vi "LVDimInterface.dim_dispatcher.vi"(2 "start":refnum<k4>, 4 "stop":refnum<k4>) -> ()   [LabVIEW 2014, in "LVDimInterface.lvlib"]
doc: "This VI should only be used, when using the DIMWrapper interface in polling mode. This VI must be started prior to any other DIM VIs. This VI must only exist once per execution system.\n\nHistory: 22-FEB-2006, Dietrich Beck\n\nCopyright (C)\nGesellschaft für Schwerionenforschung, GSI\nPlanckstr. 1\n64291 Darmstadt\nGermany\n\nContact: D.Beck@gsi.de \n\nThis program is free software; you can redistribute it and/or modify it under the terms of the \nGNU General Public License as published by the Free Software Foundation; either version 2 of the license, or (at your option) any later version.\n\nThis program is distributed in the hope that it will be useful, but WITHOUT ANY WARRANTY; without even the implied warranty of MERCHANTABILITY or FITNESS FOR A PARTICULAR PURPOSE. See the GNU General License for more details (http://www.gnu.org).\n\nGesellschaft für Schwerionenforschung, GSI\nPlanckstr. 1, 64291 Darmstadt, Germany\nFor all questions and ideas contact D. Beck.\nLast update: 16-DEC-2005"
uses:
  LVDimInterface.lvlib
  LVDimInterface.queue type.ctl
  LVDimInterface.notifier type.ctl
  bin/libDimWrapper.dll
  bin/libDimWrapper.so
  bin/libDimWrapperSPL.dll
panel:
  out "error out":errorcluster
  out "pollingMode":bool
  in  "notifierRef":T1
  out "loopCounter":i32
  in  "queueRef":T2
  out "nOfReceived":i32
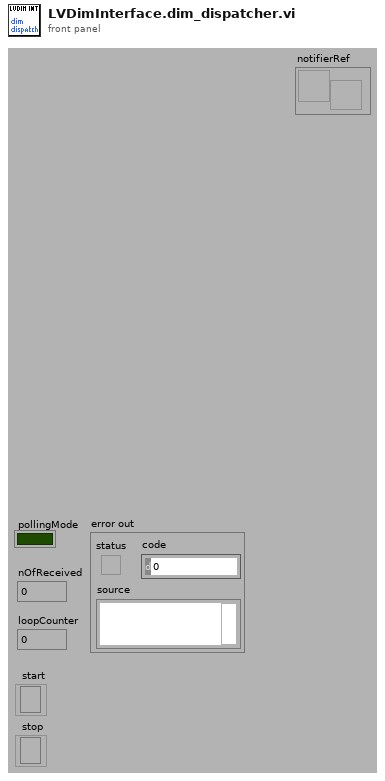
[diagram p1: front panel]
types:
  T1 = typedef "LVDimInterface.lvlib/LVDimInterface.notifier type.ctl" = refnum<notifier>
  T2 = typedef "LVDimInterface.lvlib/LVDimInterface.queue type.ctl" = refnum<queue>
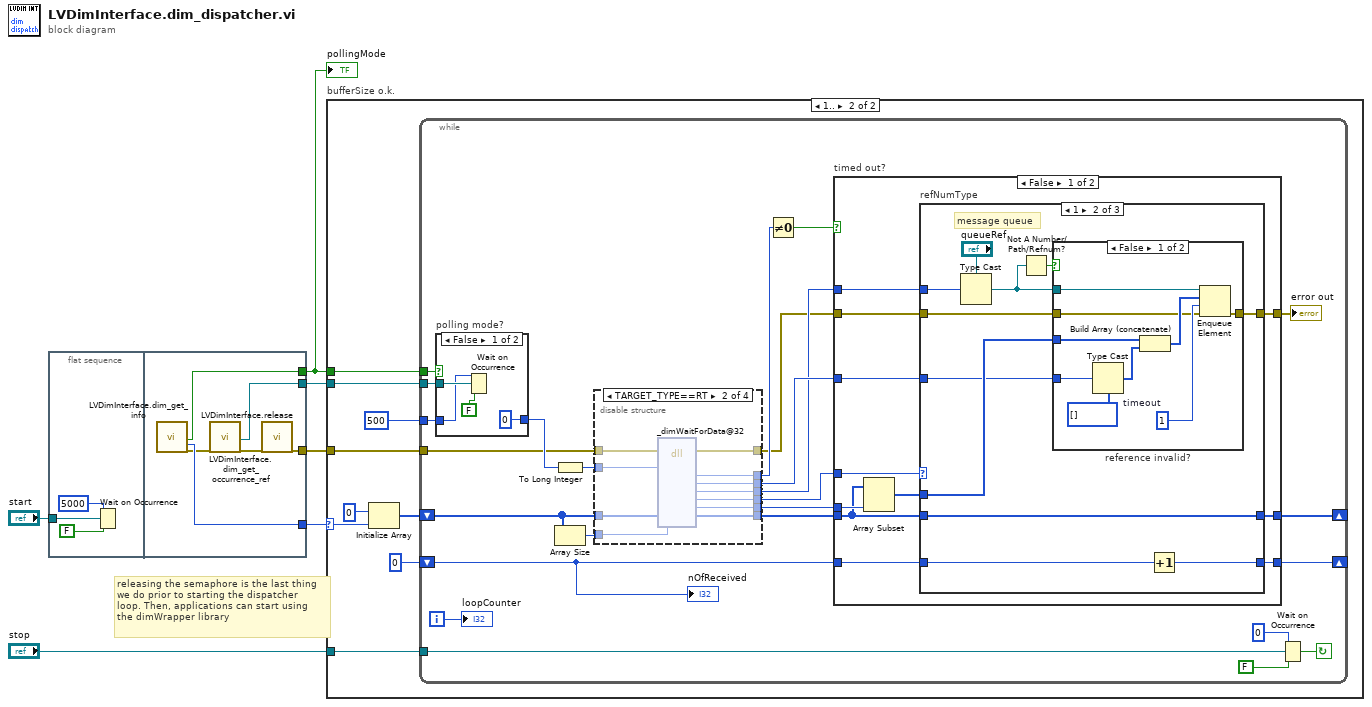
[diagram p0: block diagram]
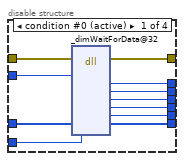
[diagram p3: hidden frame]
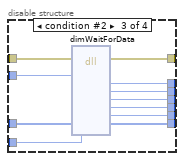
[diagram p4: hidden frame]
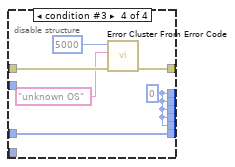
[diagram p5: hidden frame]
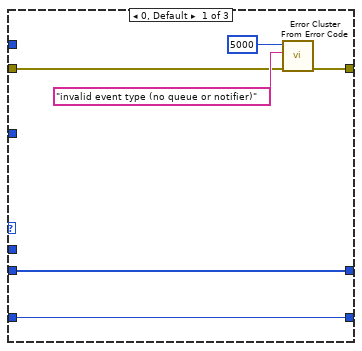
[diagram p6: hidden frame]
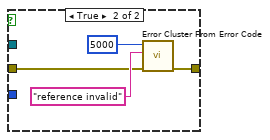
[diagram p7: hidden frame]
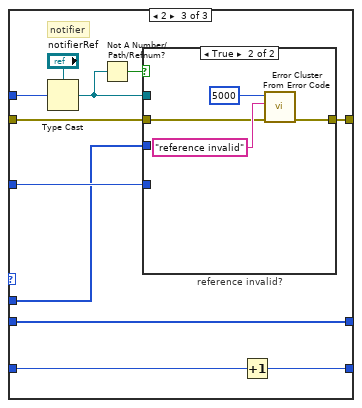
[diagram p8: hidden frame]
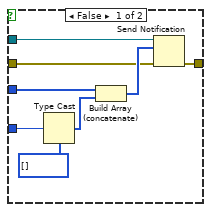
[diagram p9: hidden frame]
diagram:
  # "releasing the semaphore is the last thing\nwe do prior to starting the dispatcher\nloop. Then, applications can start using\nthe dimWrapper library"
  n1 = flat-sequence {
    tunnel: "start" -> [w9]
    tunnel: [w13] -> w2
    tunnel: [w14] -> w6
    tunnel: [w15] -> w4
    tunnel: [w11] -> w1
    frame #0 {
      n2 = Wait on Occurrence(1:FALSE ("ignore previous (T)"), 2:w9, 3:5000 ("ms timeout (-1)")) -> ()  [unwired: 1 out]
    }
    frame #1 {
      n3 = call "LVDimInterface.dim_get_info.vi"() -> ("pollingMode"=w14:bool, "maxBufferSize"=w15:i32, "error out"=w12:errorcluster)  [unwired: 13 in, 4 out]
      n4 = call "LVDimInterface.dim_get_occurrence_ref.vi"("error in (no error)"=w12) -> ("occurrence"=w13:refnum<k4>, "error out"=w10:errorcluster)  [unwired: 17 in]
      n5 = call "LVDimInterface.release.vi"("error in (no error)"=w10) -> ("error out"=w11:errorcluster)  [unwired: 18 in]
    }
  }
  n6 = case "bufferSize o.k." shown="1.." w4 {
    selector: w4 -> [_ w19]
    tunnel: w6 -> [_ w21]
    tunnel: "stop" -> [_ w18]
    tunnel: w2 -> [_ w17]
    tunnel: w1 -> [_ w16]
    frame 0, Default {
    }
    frame 1.. {
      n7 = Initialize Array(i8 0, w19) -> (w22:i8[])
      n8 = while {
        shift-right: [w48] -> _
        shift-left: 0 -> [w49]
        shift-right: [w47] -> _
        shift-left: w22 -> [w46]
        tunnel: w21 -> [w44]
        tunnel: w17 -> [w43]
        tunnel: u32 500 ("timeout") -> [w42]
        tunnel: w18 -> [w39]
        tunnel: w16 -> [w27]
        i -> [w45]
        stop <- w40 continue-if-true
        n9 = case "polling mode?" shown="False" w44 {
          tunnel: w43 -> [w159 _]
          tunnel: w42 -> [w157 w160]
          tunnel: [u32 0 ("timeout") w160] -> w41
          frame False {
            n10 = Wait on Occurrence(1:FALSE ("ignore previous (T)"), 2:w159, 3:w157) -> ()  [unwired: 1 out]
          }
          frame True {
          }
        }
        n11 = To Long Integer(number=w41) -> (32bit integer=w35:i32)
        n12 = Array Size(array=w46) -> (size(s)=w34:i32)
        n13 = disable-structure "Conditional Disable Structure" shown="TARGET_TYPE==RT" {
          disable-tunnel: [w60 w71 w82 w88] -> w36
          disable-tunnel: w35 -> [w59 w70 w81 _]
          disable-tunnel: w34 -> [w58 w69 w80 _]
          disable-tunnel: w46 -> [w57 w68 w79 w87]
          disable-tunnel: [w56 w67 w78 w87] -> w33
          disable-tunnel: [w55 w66 w77 w88] -> w31
          disable-tunnel: [w54 w65 w76 w88] -> w30
          disable-tunnel: [w53 w64 w75 w88] -> w29
          disable-tunnel: [w52 w63 w74 w88] -> w28
          disable-tunnel: w27 -> [w51 w62 w72 w86]
          disable-tunnel: [w50 w61 w73 w85] -> w26
          frame condition #0 (active) {
            n14 = dll-call lib="D:/Git/CS-framework/CSlibraries-extern/DimLVEvent/bin/libDimWrapper.dll" fn="_dimWaitForData@32" label="dimWaitForData"(error in=w51, "timeout"=w59, "copyBuffer"=w57, "copyBufferSize"=w58) -> (error out=w50:errorcluster, "timedOut"=w60:i32, "callBackID"=w53:i32, "refNum"=w52:u32, "refNumType"=w54:i32, "size"=w55:i32, "copyBuffer"=w56:i8[])  [unwired: 10 in, 1 out]
          }
          frame condition #1 {
            n15 = dll-call lib="D:/Git/CS-framework/CSlibraries/DimLVEvent/bin/libDimWrapperSPL.dll" fn="_dimWaitForData@32" label="dimWaitForData"(error in=w62, "timeout"=w70, "copyBuffer"=w68, "copyBufferSize"=w69) -> (error out=w61:errorcluster, "timedOut"=w71:i32, "callBackID"=w64:i32, "refNum"=w63:u32, "refNumType"=w65:i32, "size"=w66:i32, "copyBuffer"=w67:i8[])  [unwired: 10 in, 1 out]
          }
          frame condition #2 {
            n16 = dll-call lib="D:/Git/CS-framework/CSlibraries/DimLVEvent/bin/libDimWrapper.so" fn="dimWaitForData"(error in=w72, "timeout"=w81, "copyBuffer"=w79, "copyBufferSize"=w80) -> (error out=w73:errorcluster, "timedOut"=w82:i32, "callBackID"=w75:i32, "refNum"=w74:u32, "refNumType"=w76:i32, "size"=w77:i32, "copyBuffer"=w78:i8[])  [unwired: 10 in, 1 out]
          }
          frame condition #3 {
            w88 = 0 ("timedOut")
            n17 = call <vilib>:"Error Cluster From Error Code.vi"("error in (no error)"=w86, "error message (\"\")"="unknown OS" ("error message (\"\")"), "error code (0)"=5000) -> ("error out"=w85:errorcluster)  [unwired: 6 in]
          }
        }
        n18 = Not Equal To 0?(x=w36) -> (x != 0?=w32:bool)
        n19 = case "timed out?" shown="False" w32 {
          tunnel: w30 -> [w97 _]
          tunnel: w28 -> [w96 _]
          tunnel: w29 -> [w98 _]
          tunnel: w33 -> [w94 w154]
          tunnel: w49 -> [w92 w155]
          tunnel: [w91 w155] -> w48
          tunnel: [w93 w154] -> w47
          tunnel: w31 -> [w99 _]
          tunnel: w26 -> [w90 w153]
          tunnel: [w89 w153] -> w25
          frame False {
            n20 = Array Subset(array=w94, length=w99) -> (w95:i8[])  [unwired: 1 in]
            n21 = case "refNumType" shown="1" w97 {
              tunnel: w98 -> [_ w109 w137]
              tunnel: w96 -> [_ w110 w136]
              tunnel: w95 -> [_ w111 w135]
              tunnel: [w105 w114 w134] -> w93
              tunnel: w94 -> [w105 w114 w134]
              tunnel: [w104 w112 w132] -> w91
              tunnel: w92 -> [w104 w113 w133]
              tunnel: w90 -> [w101 w107 w131]
              tunnel: [w100 w106 w130] -> w89
              frame 0, Default {
                n22 = call <vilib>:"Error Cluster From Error Code.vi"("error in (no error)"=w101, "error message (\"\")"="invalid event type (no queue or notifier)" ("error message (\"\")"), "error code (0)"=5000) -> ("error out"=w100:errorcluster)  [unwired: 6 in]
              }
              frame 1 {
                # "message queue"
                n23 = Type Cast(type="queueRef", x=w110) -> (*(type *) &x=w115:T2)
                n24 = Not A Number/Path/Refnum?(number/path/refnum=w115) -> (NaN/Path/Refnum?=w116:bool)
                n25 = case "reference invalid?" shown="False" w116 {
                  tunnel: w111 -> [w122 _]
                  tunnel: w115 -> [w125 _]
                  tunnel: w109 -> [w124 _]
                  tunnel: w107 -> [w118 w127]
                  tunnel: [w117 w126] -> w106
                  frame False {
                    w119 = 1  # timeout
                    n26 = Type Cast(type=i8[] [] ("element"), x=w124) -> (*(type *) &x=w121:i8[])
                    n27 = Build Array (concatenate)(w122, w121) -> (w120:i8[])
                    n28 = Enqueue Element(queue=w125, element=w120, timeout in ms (-1)=w119, error in (no error)=w118) -> (error out=w117:errorcluster)  [unwired: 2 out]
                  }
                  frame True {
                    n29 = call <vilib>:"Error Cluster From Error Code.vi"("error in (no error)"=w127, "error message (\"\")"="reference invalid" ("error message (\"\")"), "error code (0)"=5000) -> ("error out"=w126:errorcluster)  [unwired: 6 in]
                  }
                }
                n30 = Increment(x=w113) -> (x+1=w112:i32)
              }
              frame 2 {
                # "notifier"
                n31 = Type Cast(type="notifierRef", x=w136) -> (*(type *) &x=w139:T1)
                n32 = Not A Number/Path/Refnum?(number/path/refnum=w139) -> (NaN/Path/Refnum?=w138:bool)
                n33 = case "reference invalid?" shown="True" w138 {
                  tunnel: w139 -> [w148 _]
                  tunnel: w137 -> [w146 _]
                  tunnel: w135 -> [w143 _]
                  tunnel: w131 -> [w142 w150]
                  tunnel: [w141 w149] -> w130
                  frame False {
                    n34 = Type Cast(type=i8[] [] ("element"), x=w146) -> (*(type *) &x=w145:i8[])
                    n35 = Build Array (concatenate)(w143, w145) -> (w144:i8[])
                    n36 = Send Notification(notification=w144, notifier=w148, error in (no error)=w142) -> (error out=w141:errorcluster)  [unwired: 1 out]
                  }
                  frame True {
                    n37 = call <vilib>:"Error Cluster From Error Code.vi"("error in (no error)"=w150, "error message (\"\")"="reference invalid" ("error message (\"\")"), "error code (0)"=5000) -> ("error out"=w149:errorcluster)  [unwired: 6 in]
                  }
                }
                n38 = Increment(x=w133) -> (x+1=w132:i32)
              }
            }
          }
          frame True {
          }
        }
        "error out" <- w25
        n39 = Wait on Occurrence(1:FALSE ("ignore previous (T)"), 2:w39, 3:0 ("ms timeout (-1)")) -> (0:w40:bool)
        "loopCounter" <- w45
        "nOfReceived" <- w49
      }
    }
  }
  "pollingMode" <- w6
